vi "MagBoard_n128_File_Quick_Analysis.vi"(8 "error in":errorcluster, 11 "Path":path) -> (0 "error out":errorcluster)   [LabVIEW 2018]
uses:
  <vilib>/Math Plots/3D Math Plots/3D Surface/3D Surface XCtrl/3D Surface.xctl
  subVIs/calibration/FGVs/FGV States.ctl
  <vilib>/Utility/file.llb/Read Delimited Spreadsheet (I64).vi
  <vilib>/Math Plots/3D Math Plots/3D Surface/3D Surface Datatype/Public/Plot Helper (Matrix).vi
  <vilib>/Math Plots/3D Math Plots/3D Surface/3D Surface Datatype/3D Surface Datatype.lvclass
panel:
  out "Filename":string
  in  "Quit":bool
  in  "Tab Control":T1(tab)
  out "Instant Response":refnum<class "3D Plot Datatype.lvclass">[](xcontrol)
  out "Pressure - Time Integral":refnum<class "3D Plot Datatype.lvclass">[](xcontrol)
  out "Time Frame":i32(slide) scale=0.0..4881.0
  out "Data Packet":string
  out "Time":u32=4294745741
  out "Lookup Indices":i32[](array[numeric])=[0, 4, 8, 12, 1, 5, 9, 13, 16, 20, 24, 28, 17, 21, 25, 29, 15, 11, 7, 3, 14, 10, 6, 2, 31, 27, 23, 19, 30, 26, 22, 18, 32, 36, 40, 44, 33, 37, 41, 45, 48, 52, 56, 60, 49, 53, 57, 61, 47, 43, 39, 35, 46, 42, 38, 34, 63, 59, 55, 51, 62, 58, 54, 50, 64, 68, 72, 76, 65, 69, 73, 77, 80, 84, 88, 92, 81, 85, 89, 93, 79, 75, 71, 67, 78, 74, 70, 66, 95, 91, 87, 83, 94, 90, 86, 82, 96, 100, 104, 108, 97, 101, 105, 109, 112, 116, 120, 124, 113, 117, 121, 125, 111, 107, 103, 99, 110, 106, 102, 98, 127, 123, 119, 115, 126, 122, 118, 114]
  out "EOF?":bool
  in  "Start Z_Threshold":dbl=0.1 format="%#_13g"
  in  "Calibration File":string="Magboard_Btod_new_calib"
  in  "Gains":dbl[](array[numeric])=[0.751, 0.751, 1.21]
  in  "Upper Limit":dbl=5.0 format="%#_13g"
  in  "Lower Limit":dbl format="%#_13g"
  out "Filesize (bytes)":i64
  out "No. Packets":dbl
  out "Calibrated Output":dbl[][](array[numeric])
  out "B xyz":dbl[][](array[numeric]) format="%#.0f"
  # "scapes: Analysis"
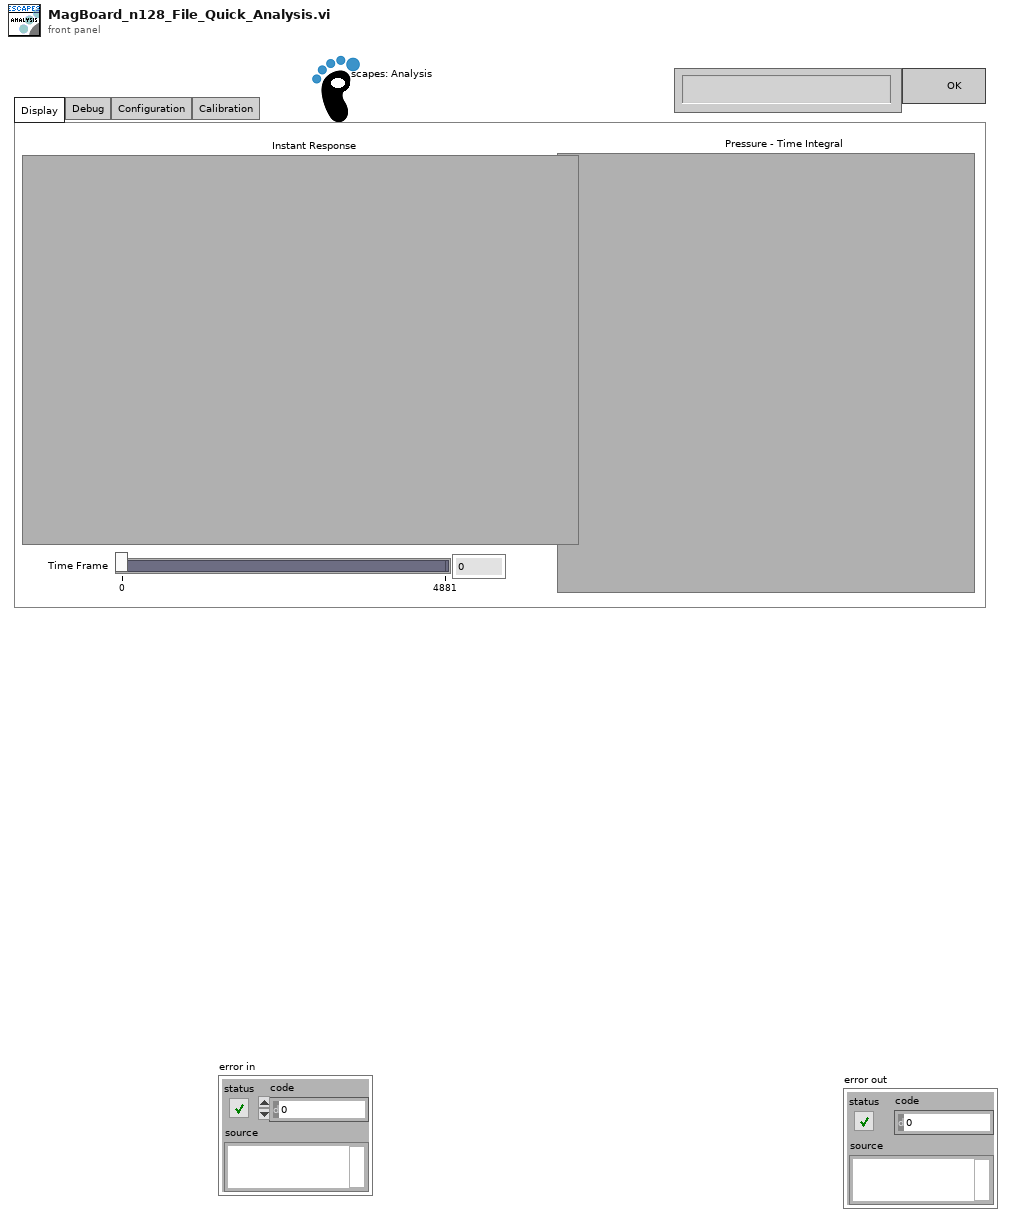
[diagram p1: front panel]
types:
  T1 = enum32{"Display", "Debug", "Configuration", "Calibration"}
  T2 = typedef "FGV States.ctl" = enum16{"Get", "Set", "Reset"}
  T3 = cluster{cluster{dbl[][], "Array":dbl[][]}, cluster{dbl[][], "Array":dbl[][]}, cluster{dbl[][], "Array":dbl[][]}, cluster{dbl[][], "Array":dbl[][]}}
  T4 = cluster{cluster{dbl[][], "Array":dbl[][]}, cluster{dbl[][], "Array":dbl[][]}, cluster{dbl[][], "Array":dbl[][]}, cluster{dbl[][], "Array":dbl[][]}}[]
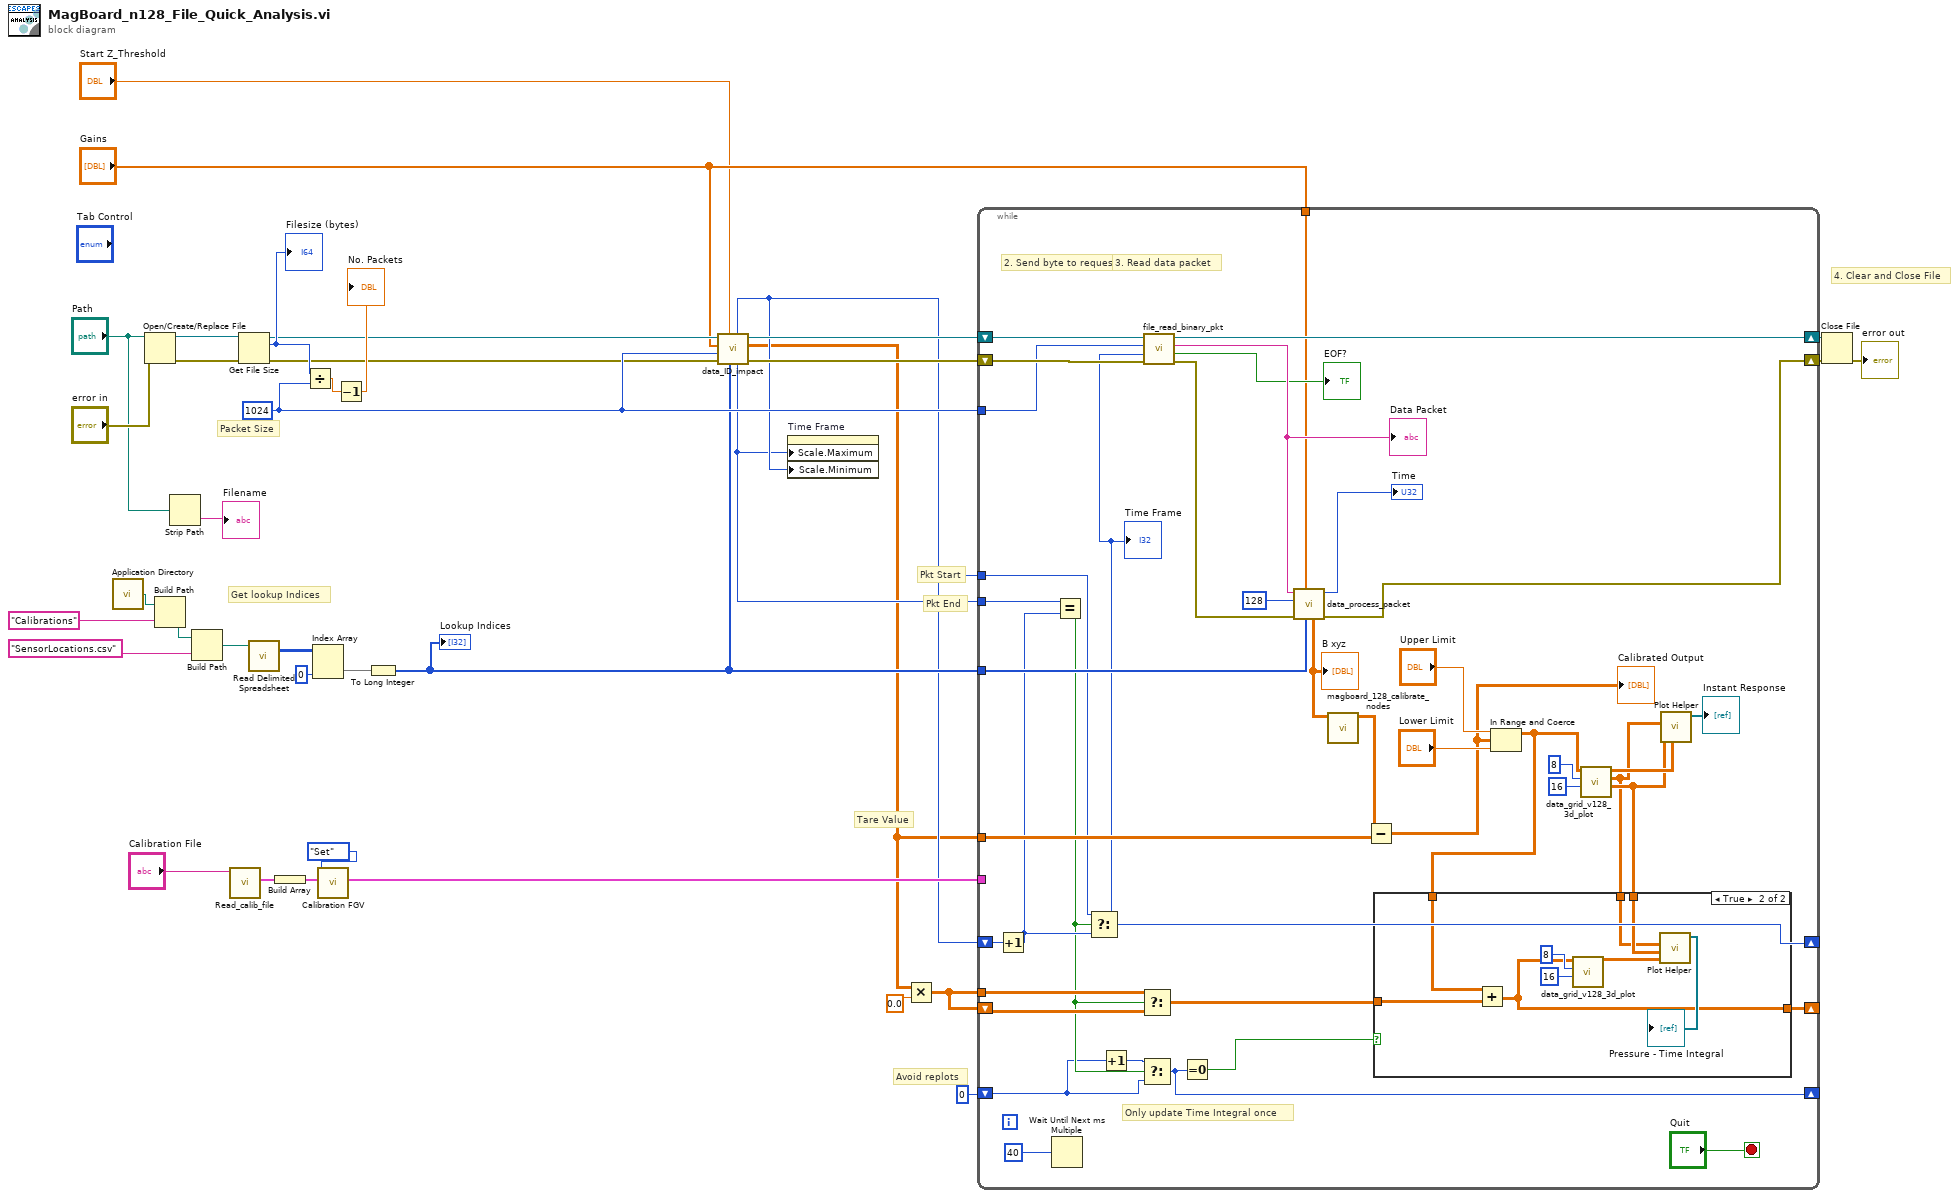
[diagram p0: block diagram]
diagram:
  w17 = 1024 ("count (1)")
  # "Tare Value"
  # "Avoid replots"
  # "Pkt End"
  # "Pkt Start"
  # "Packet Size"
  # "Get lookup Indices"
  # "4. Clear and Close File"
  n1 = call <vilib>:"Application Directory.vi"() -> ("Application Directory"=w20:path)
  n2 = Open/Create/Replace File(file path (use dialog)="Path", error in="error in") -> (refnum out=w28:refnum<file>, error out=w27:errorcluster)  [unwired: 4 in, 1 out]
  n3 = Build Path(base path=w20, name or relative path="Calibrations" ("string")) -> (appended path=w22:path)
  n4 = Strip Path(path="Path") -> (name=→"Filename":string)  [unwired: 1 out]
  n5 = Build Path(base path=w22, name or relative path="SensorLocations.csv" ("string")) -> (appended path=w19:path)
  n6 = call "Read_calib_file.vi"("string"="Calibration File") -> ("output cluster"=w35:T3)  [unwired: 6 in, 4 out]
  n7 = Get File Size(file=w28, error in=w27) -> (refnum out=w16:refnum<file>, size (in bytes)=w25:i64, 0:w9:errorcluster)
  "Filesize (bytes)" <- w25
  n8 = call-poly <vilib>:"Read Delimited Spreadsheet.vi"("file path (dialog if empty)"=w19) -> ("all rows"=w38:i64[][])  [unwired: 9 in, 5 out]
  n9 = Build Array(w35) -> (w34:T4)
  n10 = Divide(x=w25, y=w17) -> (x/y=w26:dbl)
  n11 = Index Array(array=w38, index (col)=0 ("disabled index (col)")) -> (element=w36:i64[])  [unwired: 1 in]
  n12 = call "Calibration FGV.vi"("Calib in"=w34, "FGV States"=FGV_States."Set") -> ("Calib in 2"=w32:T4)  [unwired: 9 in]
  n13 = Decrement(x=w26) -> (x-1=→"No. Packets":dbl)
  n14 = To Long Integer(number=w36) -> (32bit integer=w12:i32[])
  "Lookup Indices" <- w12
  n15 = call "data_ID_impact.vi"("Sensor Lookup Indices"=w12, "Start Z_Threshold"="Start Z_Threshold", "error in (no error)"=w9, "Pkt Size"=w17, "Gains"="Gains", "Byte Stream File in"=w16) -> ("error out"=w14:errorcluster, "Sensor_Tare"=w5:dbl[][], "Byte Stream File out"=w15:refnum<file>, "N_end"=w7:i32, "N_start"=w8:i32)  [unwired: 1 in]
  n16 = property on="Time Frame" class="Slide (strict)"("Scale.Maximum"=w7, "Scale.Minimum"=w8) -> ()  [unwired: 2 in, 2 out]
  n17 = Multiply(x=w5, y=0.0 ("Playback dT")) -> (x*y=w4:dbl[][])
  n18 = while {
    shift-right: [w72] -> w30
    shift-left: w15 -> [w74]
    tunnel: w12 -> [w78]
    shift-right: [w76] -> w31
    shift-left: w14 -> [w73]
    tunnel: w32 -> [_]
    tunnel: w17 -> [w67]
    tunnel: "Gains" -> [w59]
    tunnel: w5 -> [w61]
    tunnel: w8 -> [w54]
    tunnel: w7 -> [w58]
    shift-right: [w53] -> _
    shift-left: w8 -> [w56]
    shift-right: [w51] -> _
    shift-left: w4 -> [w47]
    tunnel: w4 -> [w48]
    shift-right: [w40] -> _
    shift-left: u32 0 ("Playback dT") -> [w41]
    stop <- "Quit" stop-if-true
    # "Only update Time Integral once"
    # "3. Read data packet"
    # "2. Send byte to request reading"
    n19 = Increment(x=w56) -> (x+1=w55:i32)
    n20 = Wait Until Next ms Multiple(millisecond multiple=u32 40 ("Playback dT")) -> ()  [unwired: 1 out]
    n21 = Equal?(x=w58, y=w55) -> (x = y?=w43:bool)
    n22 = Select(t=w54, s=w43, f=w55) -> (s? t:f=w53:i32)
    "Time Frame" <- w53
    n23 = Increment(x=w41) -> (x+1=w42:u32)
    n24 = Select(t=w48, s=w43, f=w47) -> (s? t:f=w46:dbl[][])
    n25 = Select(t=w42, s=w43, f=w41) -> (s? t:f=w40:u32)
    n26 = call "file_read_binary_pkt.vi"("error in (no error)"=w73, "Packet No."=w53, "Pkt Size(bytes)"=w67, "Byte Stream File in"=w74) -> ("error out"=w71:errorcluster, "EOF?"=→"EOF?":bool, "Packet"=w68:string, "Byte Stream File out"=w72:refnum<file>)  [unwired: 4 in]
    "Data Packet" <- w68
    n27 = Equal To 0?(x=w40) -> (x = 0?=w39:bool)
    n28 = call "data_process_packet.vi"("Sensor Lookup Indices"=w78, "Gains"=w59, "error in (no error)"=w71, "No. Sensors"=128 ("No. Nodes"), "Binary Input Data"=w68) -> ("error out"=w76:errorcluster, "Time"=→"Time":u32, "Sensors (uT)"=w75:dbl[][])  [unwired: 2 in, 2 out]
    "B xyz" <- w75
    n29 = call "magboard_128_calibrate_nodes.vi"("Sensor Input (mT)"=w75) -> ("Sensor Output - Position (mm)"=w63:dbl[][])  [unwired: 10 in]
    n30 = Subtract(x=w63, y=w61) -> (x-y=w52:dbl[][])
    "Calibrated Output" <- w52
    n31 = In Range and Coerce(upper limit="Upper Limit", x=w52, lower limit="Lower Limit") -> (coerced(x)=w44:dbl[][])  [unwired: 1 out]
    n32 = call "data_grid_v128_3d_plot.vi"("No. Rows"=16 ("Row Length"), "No. Columns"=8, "Sensor Data"=w44) -> ("Y (GRID)"=w50:dbl[][], "X (GRID)"=w49:dbl[][], "Z (GRID)"=w64:dbl[][])  [unwired: 6 in]
    n33 = case shown="True" w39 {
      tunnel: [w80 w86] -> w51
      tunnel: w50 -> [_ w84]
      tunnel: w49 -> [_ w83]
      tunnel: w46 -> [w80 w82]
      tunnel: w44 -> [_ w81]
      frame False {
      }
      frame True {
        n34 = Add(x=w81, y=w82) -> (x+y=w86:dbl[][])
        n35 = call "data_grid_v128_3d_plot.vi"("No. Rows"=16 ("Row Length"), "No. Columns"=8, "Sensor Data"=w86) -> ("Z (GRID)"=w85:dbl[][])  [unwired: 6 in, 2 out]
        n36 = call-poly <vilib>:"Plot Helper.vi"("z matrix"=w85, "y matrix"=w84, "x matrix"=w83) -> ("3D Plot lvclass Array out"=→"Pressure - Time Integral":refnum<class "3D Plot Datatype.lvclass">[])  [unwired: 3 in, 5 out]
      }
    }
    n37 = call-poly <vilib>:"Plot Helper.vi"("z matrix"=w64, "y matrix"=w50, "x matrix"=w49) -> ("3D Plot lvclass Array out"=→"Instant Response":refnum<class "3D Plot Datatype.lvclass">[])  [unwired: 3 in, 5 out]
  }
  n38 = Close File(refnum=w30, error in=w31) -> (error out=→"error out":errorcluster)  [unwired: 1 out]
